vi "Host-Convert-SGL-to-FXP.vi"(11 "Complex Data (in)":csg[](array[numeric])=[0.0+1.0i, 1.0+2.0i, 3.0+0.55i, 0.0+0.0i, 0.0+1.0i, 1.0+2.0i, 3.0+0.55i, 0.0+0.0i]) -> (2 "[FPGA] Array Size":u64, 3 "Complex Data Ready for FPGA (out)":u64[](array[numeric]))   [LabVIEW 2014]
panel:
  out "Real SGL(out)":sgl[](array[numeric])
  out "Real FXP (in)":fxp<+/-,24,7>[](array[numeric])
  out "Imag FXP (in)":fxp<+/-,24,7>[](array[numeric])
  out "Imag SGL (out)":sgl[](array[numeric])
  out "Imag FXP (out)":fxp<+/-,32,7>[](array[numeric])
  out "Real FXP (out)":fxp<+/-,32,7>[](array[numeric])
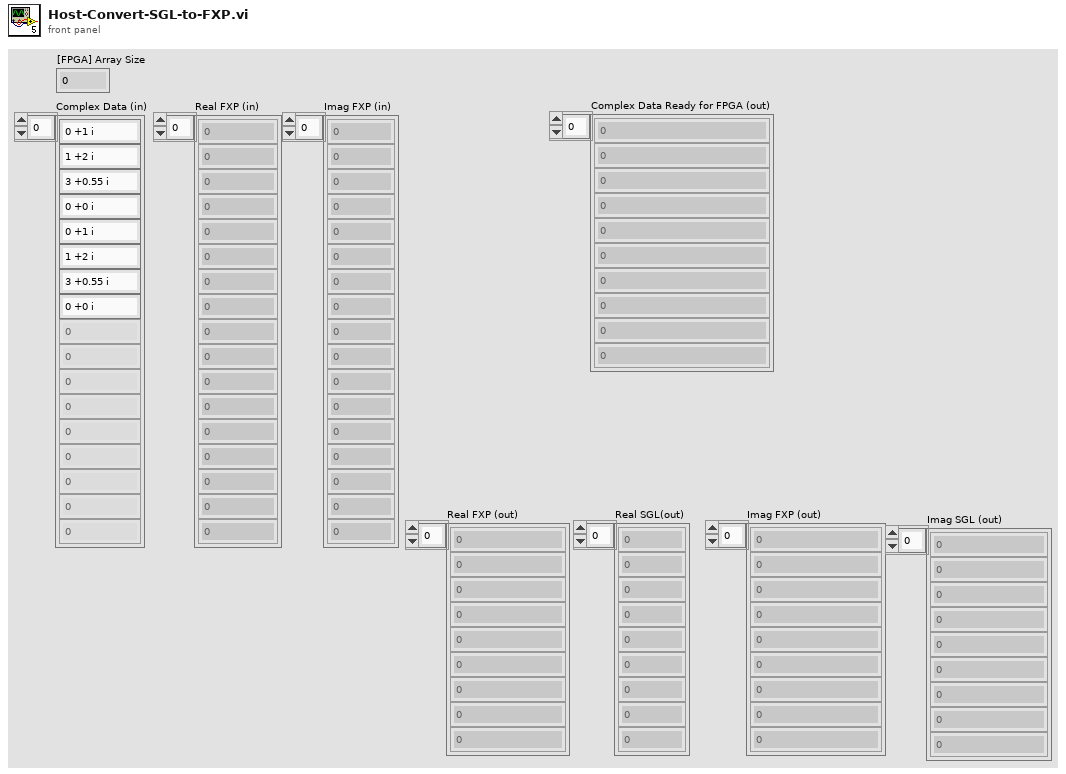
[diagram p1: front panel]
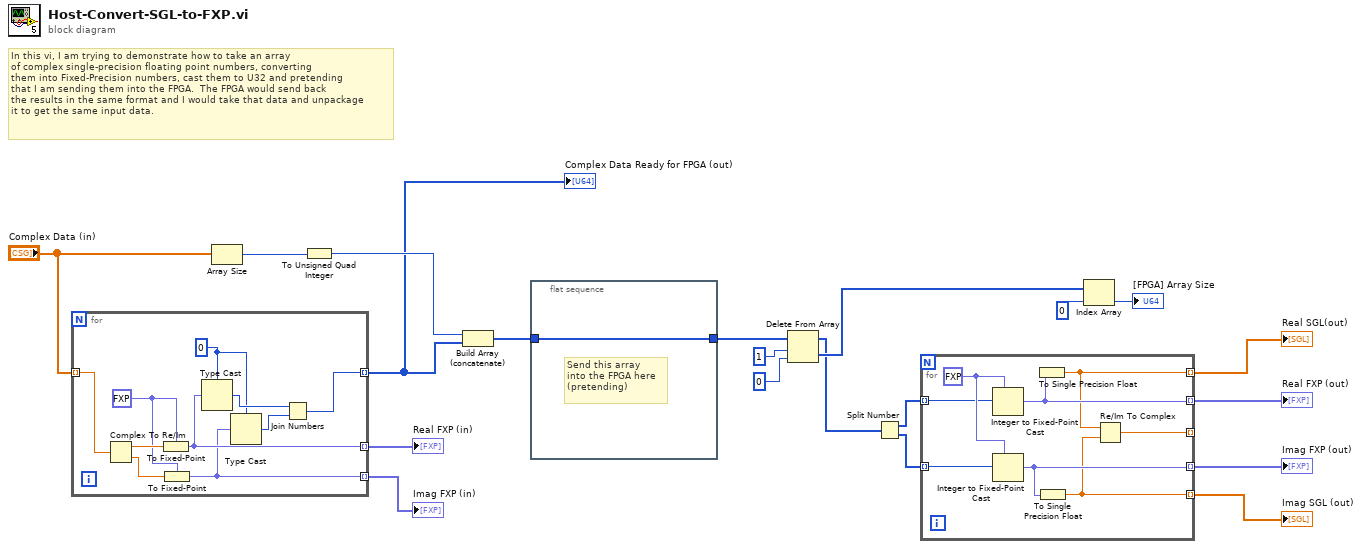
[diagram p0: block diagram]
diagram:
  # "In this vi, I am trying to demonstrate how to take an array\nof complex single-precision floating point numbers, converting\nthem into Fixed-Precision numbers, cast them to U32 and pretending\nthat I am sending them into the FPGA.  The FPGA would send back\nthe results in the same format and I would take that data and unpackage\nit to get the same input data."
  n1 = for {
    tunnel: "Complex Data (in)" -> [w30] mode=indexing
    tunnel: [w21] -> w2 mode=indexing
    tunnel: [w26] -> w7 mode=indexing
    tunnel: [w25] -> w6 mode=indexing
    w22 = u32 0
    w27 = fxp<+/-,24,7> 0.0 ("real data in")
    n2 = Complex To Re/Im(x + iy=w30) -> (x=w29:sgl, y=w28:sgl)
    n3 = To Fixed-Point(fixed-point type=w27, number=w29) -> (fixed-point=w26:fxp<+/-,24,7>)
    n4 = To Fixed-Point(fixed-point type=w27, number=w28) -> (fixed-point=w25:fxp<+/-,24,7>)
    n5 = Type Cast(type=w22, x=w26) -> (*(type *) &x=w24:u32)
    n6 = Type Cast(type=w22, x=w25) -> (*(type *) &x=w23:u32)
    n7 = Join Numbers(hi=w24, lo=w23) -> ((hi.lo)=w21:u64)
  }
  "Imag FXP (in)" <- w6
  "Real FXP (in)" <- w7
  "Complex Data Ready for FPGA (out)" <- w2
  n8 = Array Size(array="Complex Data (in)") -> (size(s)=w19:i32)
  n9 = To Unsigned Quad Integer(1:w19) -> (0:w18:u64)
  n10 = Build Array (concatenate)(w18, w2) -> (w3:u64[])
  n11 = flat-sequence {
    tunnel: [w31] -> w4
    tunnel: w3 -> [w31]
    frame #0 {
      # "Send this array\ninto the FPGA here\n(pretending)"
    }
  }
  n12 = Delete From Array(array=w4, length=1 ("index"), index=0) -> (deleted portion=w16:u64[], array with subset deleted=w1:u64[])
  n13 = Split Number(x=w1) -> (hi(x)=w12:u32[], lo(x)=w9:u32[])
  n14 = for {
    tunnel: w12 -> [w37] mode=indexing
    tunnel: w9 -> [w38] mode=indexing
    tunnel: [w36] -> w10 mode=indexing
    tunnel: [w35] -> w11 mode=indexing
    tunnel: [w33] -> w8 mode=indexing
    tunnel: [w34] -> w5 mode=indexing
    tunnel: [w32] -> _ mode=indexing
    w39 = fxp<+/-,32,7> 0.0 ("real data in")
    n15 = Integer to Fixed-Point Cast(fixed-point type=w39, integer=w37) -> (fixed-point=w35:fxp<+/-,32,7>)
    n16 = Integer to Fixed-Point Cast(fixed-point type=w39, integer=w38) -> (fixed-point=w36:fxp<+/-,32,7>)
    n17 = To Single Precision Float(number=w35) -> (single precision float=w34:sgl)
    n18 = To Single Precision Float(number=w36) -> (single precision float=w33:sgl)
    n19 = Re/Im To Complex(1:w33, 2:w34) -> (0:w32:csg)
  }
  "Real FXP (out)" <- w11
  "Imag FXP (out)" <- w10
  "Imag SGL (out)" <- w8
  "Real SGL(out)" <- w5
  n20 = Index Array(array=w16, index=0) -> (element=→"[FPGA] Array Size":u64)
